vi "Convert64BitTo4Channels.vi"(10 "64 Bit Int":u64, 11 "Scale Factor":dbl) -> (0 "Channel 3":dbl, 1 "Channel 2":dbl, 2 "Channel 1":dbl, 3 "Channel 0":dbl)   [LabVIEW 2014]
panel:
  out "Channel 4":dbl
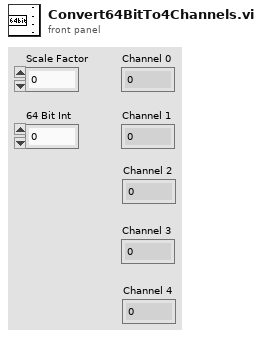
[diagram p1: front panel]
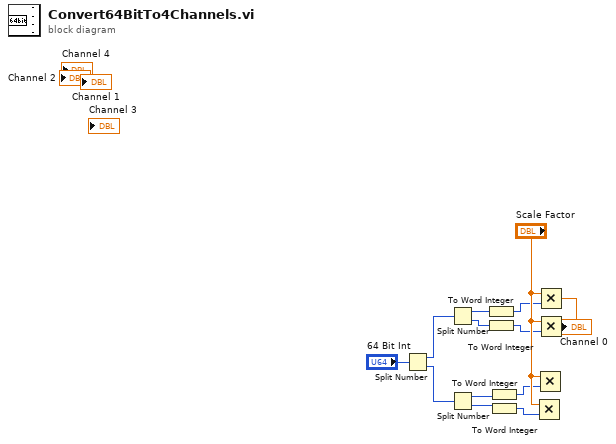
[diagram p0: block diagram]
diagram:
  n1 = Split Number(x="64 Bit Int") -> (hi(x)=w2:u32, lo(x)=w3:u32)
  n2 = Split Number(x=w2) -> (hi(x)=w4:u16, lo(x)=w7:u16)
  n3 = Split Number(x=w3) -> (hi(x)=w11:u16, lo(x)=w12:u16)
  n4 = To Word Integer(number=w4) -> (16bit integer=w5:i16)
  n5 = To Word Integer(number=w7) -> (16bit integer=w8:i16)
  n6 = To Word Integer(number=w11) -> (16bit integer=w9:i16)
  n7 = To Word Integer(number=w12) -> (16bit integer=w10:i16)
  n8 = Multiply(x="Scale Factor", y=w10) -> ()  [unwired: 1 out]
  n9 = Multiply(x="Scale Factor", y=w9) -> ()  [unwired: 1 out]
  n10 = Multiply(x="Scale Factor", y=w5) -> (x*y=→"Channel 0":dbl)
  n11 = Multiply(x="Scale Factor", y=w8) -> ()  [unwired: 1 out]
